vi "Error Reported.vi"(4 "DQMH_ARG":T1, 6 "Boolean":bool, 8 "error in":errorcluster, 9 "Additional Information":string, 10 "Error":errorcluster) -> (0 "error out":errorcluster)   [LabVIEW 2025, in "Full User Interface.lvlib"]
doc: "Send the Error Reported event to any VI registered to listen to events from the owning module.\n_____\nBased on DQMH Project Template 7.0.1.1316."
uses:
  Full User Interface.lvlib
  Error Reported Argument--cluster.ctl
  <vilib>/Delacor/Delacor QMH/Libraries/Message Queue_class/Delacor_lib_QMH_Message Queue.lvclass
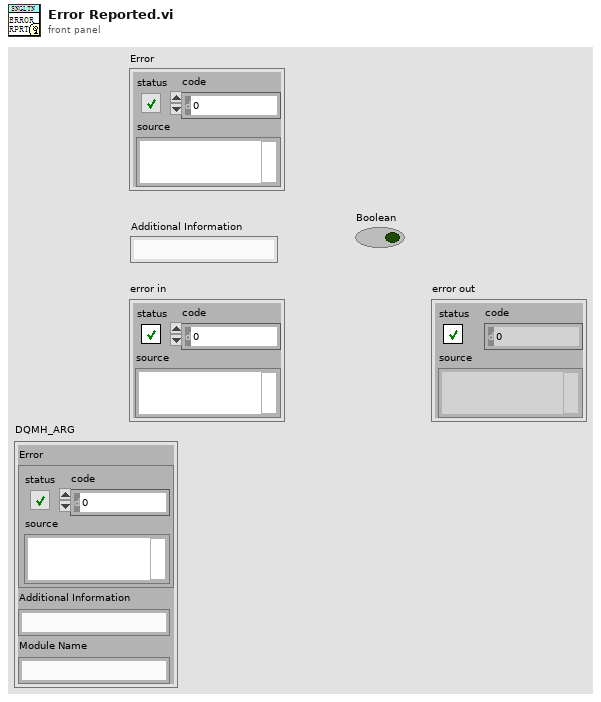
[diagram p1: front panel]
types:
  T1 = typedef "Full User Interface.lvlib/Error Reported Argument--cluster.ctl" = cluster{"Error":errorcluster, "Additional Information":string, "Module Name":string}
  T2 = typedef "Full User Interface.lvlib/Broadcast Events--cluster.ctl" = cluster{"Module Did Init":refnum<user-event>, "Status Updated":refnum<user-event>, "Error Reported":refnum<user-event>, "Module Did Stop":refnum<user-event>, "Update Module Execution Status":refnum<user-event>}
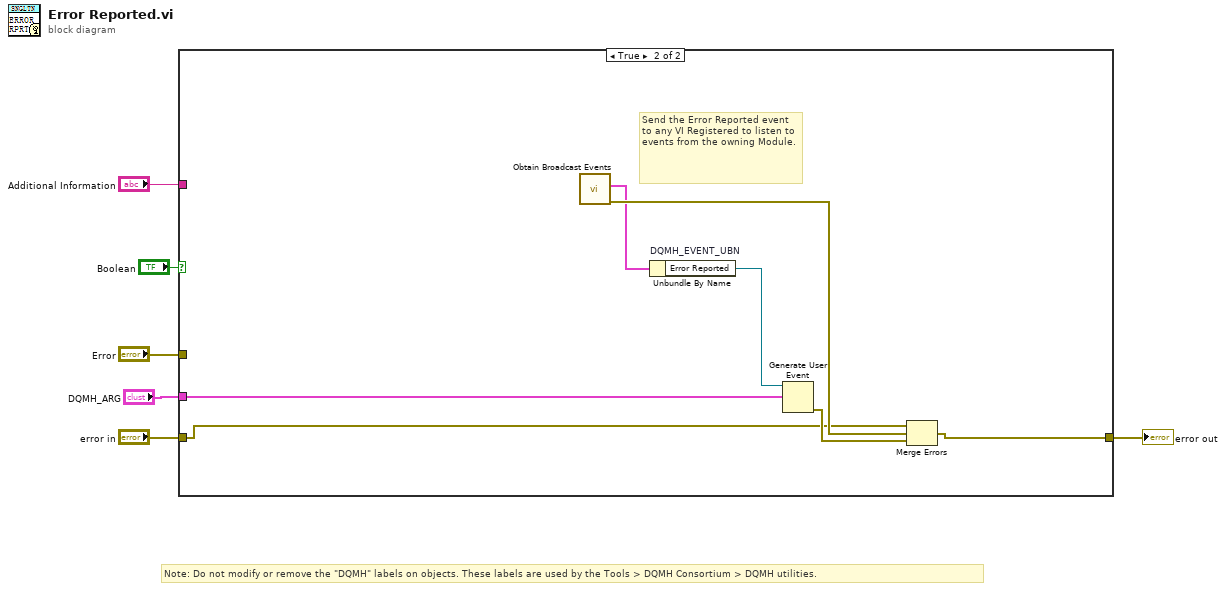
[diagram p0: block diagram]
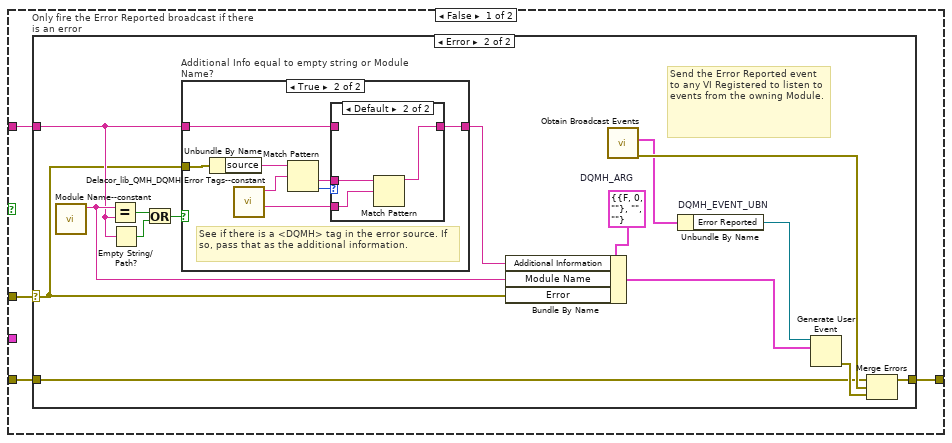
[diagram p2: hidden frame]
diagram:
  # "Note: Do not modify or remove the \"DQMH\" labels on objects. These labels are used by the Tools > DQMH Consortium > DQMH utilities."
  n1 = case shown="True" "Boolean" {
    tunnel: [w10 w40] -> w6
    tunnel: "error in" -> [w9 w41]
    tunnel: "Additional Information" -> [w8 _]
    tunnel: "Error" -> [w7 _]
    tunnel: "DQMH_ARG" -> [_ w42]
    frame False {
      n2 = case "Only fire the Error Reported broadcast if there is an error" shown="Error" w7 {
        selector: w7 -> [_ w14]
        tunnel: [w11 w26] -> w10
        tunnel: w9 -> [w11 w12]
        tunnel: w8 -> [_ w16]
        frame No Error {
          # "No error was wired in, so don't fire the Error Reported broadcast."
        }
        frame Error {
          w22 = T1 {"Error"={"status"=FALSE, "code"=0, "source"=""}, "Additional Information"="", "Module Name"=""}  # DQMH_ARG
          # "Send the Error Reported event to any VI Registered to listen to events from the owning Module."
          n3 = call "Module Name--constant.vi"() -> ("Module Name"=w20:string)  [unwired: 11 in]
          n4 = Equal?(x=w20, y=w16) -> (x = y?=w19:bool)
          n5 = Empty String/Path?(string/path=w16) -> (empty?=w18:bool)
          n6 = Or(x=w19, y=w18) -> (x .or. y?=w17:bool)
          n7 = case "Additional Info equal to empty string or Module Name?" shown="True" w17 {
            tunnel: w16 -> [w27 w28]
            tunnel: [w27 w29] -> w15
            tunnel: w14 -> [_ w35]
            frame False {
              # "If the additional information string is not equal to empty string or module name, then the user has specified a custom string, and we should pass that value."
            }
            frame True {
              # "See if there is a <DQMH> tag in the error source. If so, pass that as the additional information."
              n8 = Unbundle By Name(w35) -> ("source"=w34:string)
              n9 = call <vilib>:"Delacor_lib_QMH_DQMH Error Tags--constant.vi"() -> ("Close Tag"=w30:string, "Open Tag"=w33:string)  [unwired: 10 in]
              n10 = Match Pattern(string=w34, regular expression=w33) -> (after substring=w31:string, offset past match=w32:i32)  [unwired: 1 in, 2 out]
              n11 = case shown="Default" w32 {
                tunnel: w31 -> [_ w39]
                tunnel: w30 -> [_ w38]
                tunnel: [w36 w37] -> w29
                tunnel: w28 -> [w36 _]
                frame -1 {
                }
                frame Default {
                  n12 = Match Pattern(string=w39, regular expression=w38) -> (before substring=w37:string)  [unwired: 1 in, 3 out]
                }
              }
            }
          }
          n13 = Bundle By Name(cluster=w22, "Additional Information"=w15, "Module Name"=w20, "Error"=w14) -> (w21:T1)
          n14 = call "Obtain Broadcast Events.vi"() -> ("error out"=w25:errorcluster, "Full User Interface Broadcast Events"=w24:T2)  [unwired: 10 in]
          n15 = Unbundle By Name "DQMH_EVENT_UBN"(w24) -> ("Error Reported"=w23:refnum<user-event>)
          n16 = Generate User Event(user event=w23, event data cluster=w21) -> (error out=w13:errorcluster)  [unwired: 2 in, 1 out]
          n17 = Merge Errors(w12, w25, w13) -> (w26:errorcluster)
        }
      }
    }
    frame True {
      # "Send the Error Reported event to any VI Registered to listen to events from the owning Module."
      n18 = call "Obtain Broadcast Events.vi"() -> ("error out"=w46:errorcluster, "Full User Interface Broadcast Events"=w45:T2)  [unwired: 10 in]
      n19 = Unbundle By Name "DQMH_EVENT_UBN"(w45) -> ("Error Reported"=w44:refnum<user-event>)
      n20 = Generate User Event(user event=w44, event data cluster=w42) -> (error out=w43:errorcluster)  [unwired: 2 in, 1 out]
      n21 = Merge Errors(w41, w46, w43) -> (w40:errorcluster)
    }
  }
  "error out" <- w6
